vi "R30-Fpga.vi"() -> ()   [LabVIEW 2015]
uses:
  <vilib>/eio/EIONode/EIONode.xnode
  <vilib>/eio/EIOMethodNode/EIOMethodNode.xnode
  <vilib>/LabVIEW Targets/FPGA/cRIO/shared/nicrio_ModuleControls/nicrio_cRIO-9871_DataBitsEnum.ctl
  <vilib>/LabVIEW Targets/FPGA/cRIO/shared/nicrio_ModuleControls/nicrio_cRIO-9871_ParityEnum.ctl
  <vilib>/eio/EIOPropertyNode/EIOPropertyNode.xnode
  <vilib>/LabVIEW Targets/FPGA/cRIO/shared/nicrio_ModuleControls/nicrio_cRIO-9871_StopBitsEnum.ctl
  <vilib>/LabVIEW Targets/FPGA/cRIO/shared/nicrio_ModuleControls/nicrio_cRIO-9871_BaudRateEnum.ctl
  <vilib>/rvi/Analysis/measure/dc-rms/XNode/niFpgaDC-RMS.xnode
  <vilib>/rvi/eio/common/nirviEmuTemplateMethod_errors.vi
  <vilib>/Platform/TimedLoop/XDataNode/wakeup.ctl
  <vilib>/Platform/TimedLoop/XDataNode/XDNodeRunTimeDep.lvlib
  <vilib>/Platform/TimedLoop/XDataNode/nitl_modes.ctl
  <vilib>/Platform/TimedLoop/XDataNode/timing_clust.ctl
  <vilib>/Platform/TimedLoop/XDataNode/XDataNode.xnode
  <vilib>/rvi/FXPMathLib/basic elements/FxpIntAccumulator/XNode/nifxpmath_IntAccumulator.xnode
  <vilib>/rvi/FXPMathLib/FxpMul/XNode/nifxpmath_Multiplier.xnode
  <vilib>/rvi/Analysis/common/codeGenErrors/XNode/niFpgaXNodeCodeGenErrorHandle.vi
  <vilib>/rvi/FXPMathLib/basic elements/FxpIntAccumulator/simVIs/DllFxpIntAccumulator_sub.vi
  <vilib>/rvi/FXPMathLib/basic elements/FxpIntAccumulator/subVIs/nifxpmath_IntAccumulator_SimConfig.ctl
  <vilib>/rvi/FXPMathLib/sim/FxpSim.dll
  <vilib>/rvi/eio/common/nirviEmuTemplatePropertyGet_errors.vi
  <vilib>/rvi/eio/common/nirviEmuTemplatePropertyGet_noerrors.vi
  <vilib>/rvi/eio/common/nirviEmuTemplatePropertySet_errors.vi
  <vilib>/rvi/eio/common/nirviEmuTemplatePropertySet_noerrors.vi
  <vilib>/LabVIEW Targets/FPGA/cRIO/shared/nicrio_ModuleControls/nicrio_cRIO-9871_LineStateEnum.ctl
panel:
  out "analog readback":fxp<+/-,26,5>[](array[numeric]) format="%.23g"
  out "switch image ion gauge":u8[](array[numeric])
  out "Time since repurge":u8[](array[numeric])
  out "1st stage temp(k)":u8[](array[numeric])
  out "2nd stage":u8[](array[numeric])
  out "Time since pump on":u8[](array[numeric])
  out "Pump On":u8[](array[numeric])
  out "R30 ESA Convectron  1":u8[](array[numeric])
  out "R30 ESA Ion gauge 1":u8[](array[numeric])
  out "R30 Detector Convectron  1":u8[](array[numeric])
  out "R30 Detector Ion gauge 1":u8[](array[numeric])
  in  "y steerer magnet":fxp<+/-,20,5> format="%.17g"
  in  "analog output":fxp<+/-,64,32>[](array[numeric])=[0.0, 0.0, 0.0, 0.0, 0.0, 0.0, 0.0]
  out "Switch Ap IN":bool
  out "Switch Ap OUT2":bool
  out "Det Ap OUT":bool
  out "Det Ap IN":bool
  out "Detector  FC IN":bool
  out "Detector FC OUT":bool
  out "Switch magnet FC OUT":bool
  out "Switch magnet FC IN":bool
  in  "Switch magnet ap":bool
  in  "Detector AP":bool
  in  "Detector FC":bool
  in  "Switch magnet FC":bool
  out "Timed Out":bool
  out "Switch object tesla meter":u8[](array[numeric])
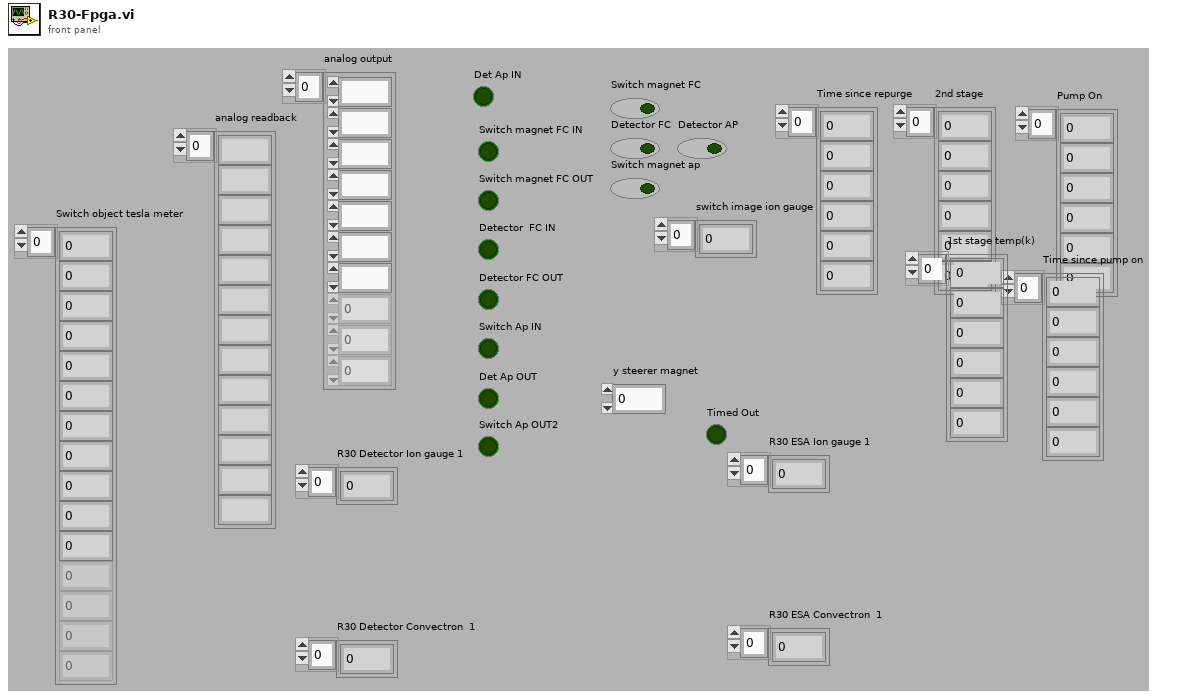
[diagram p1: front panel]
types:
  T1 = typedef "nicrio_cRIO-9871_StopBitsEnum.ctl" = enum8{"1", "1.5", "2"}
  T2 = typedef "nicrio_cRIO-9871_ParityEnum.ctl" = enum8{"None", "Odd", "Even", "Mark", "Space"}
  T3 = typedef "nicrio_cRIO-9871_DataBitsEnum.ctl" = enum8{"5", "6", "7", "8"}
  T4 = typedef "nicrio_cRIO-9871_BaudRateEnum.ctl" = enum16{"75 bps", "110 bps", "134 bps", "150 bps", "300 bps", "600 bps", "1200 bps", "1800 bps", "2400 bps", "4800 bps", "7200 bps", "9600 bps", "14.4 kbps", "19.2 kbps", "28.8 kbps", "38.4 kbps", "57.6 kbps", "115.2 kbps", "230.4 kbps", "460.8 kbps", "921.6 kbps"}
  T5 = typedef "XDNodeRunTimeDep.lvlib/timing_clust.ctl" = cluster{"Expected End [f-1]":u64, "Actual End [f-1]":u64, "Finished Late? [f-1]":bool, "Expected End [i-1]":u64, "Actual End [i-1]":u64, "Finished Late? [i-1]":bool, "Expected Start [i]":u64, "Actual Start [i]":u64, "Expected Start [f]":u64, "Actual Start [f]":u64, "Source Name":string, "Structure Name":string, "Period":i64, "Deadline":i64, "Offset":i64, "Start":i64, "Priority":i32, "Timeout":i32, "Mode":T6, "Wakeup Reason":T7, "Error":errorcluster, "Source Type":string, "Secondary Source Type":string, "Global End Time":u64, "Global Start Time":u64, "Frame Duration":u64, "Iteration Duration":u64, "Assigned CPU":i32, "I/O Scan Engine Mode":u32}
  T6 = typedef "XDNodeRunTimeDep.lvlib/nitl_modes.ctl" = enum32{"No Change", "Process missed periods, maintain original phase", "Discard missed periods, maintain original phase", "Process missed periods, ignore original phase", "Discard missed periods, ignore original phase"}
  T7 = typedef "XDNodeRunTimeDep.lvlib/wakeup.ctl" = enum32{"Normal", "Aborted", "Asynchronous wakeup", "Timing source error", "Timed loop error", "Timeout"}
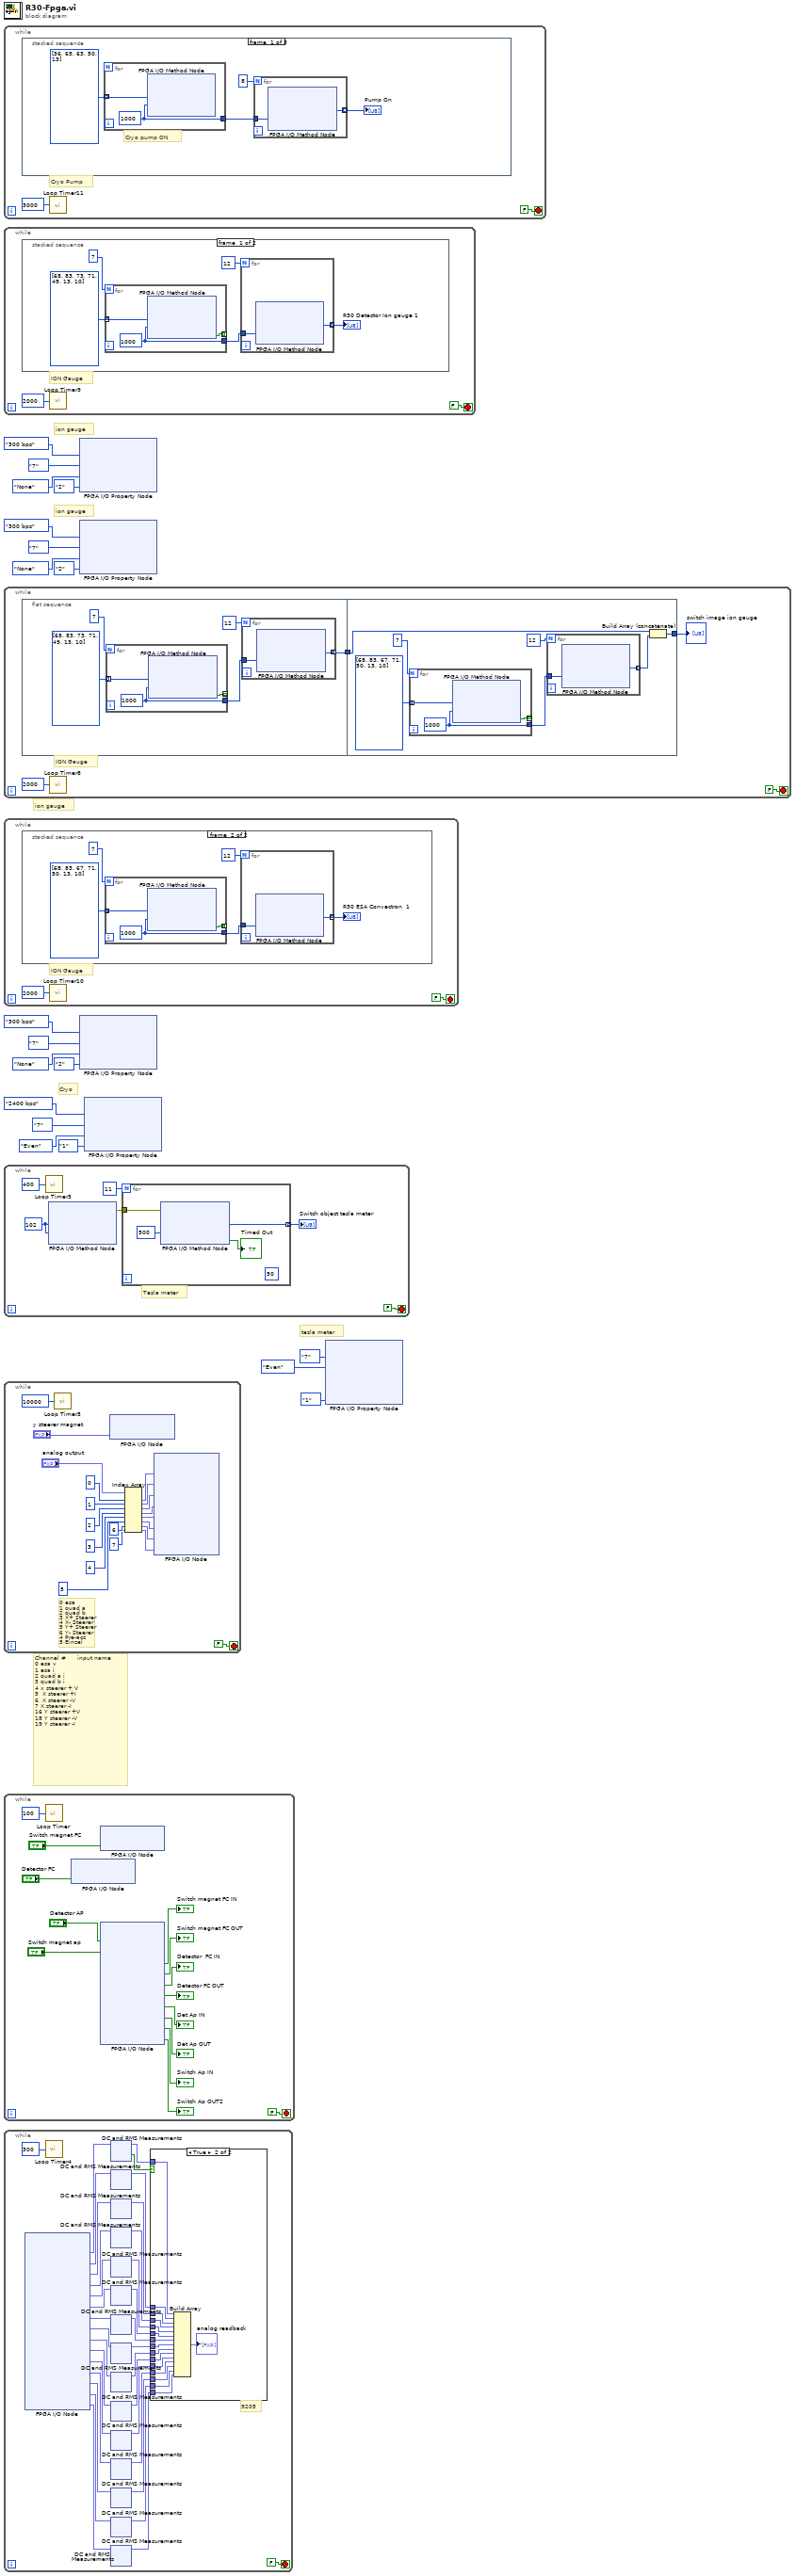
[diagram p0: block diagram]
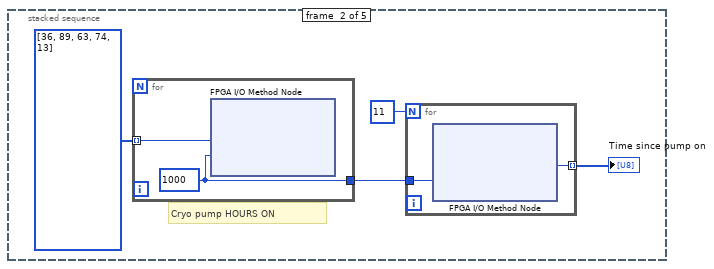
[diagram p2: hidden frame]
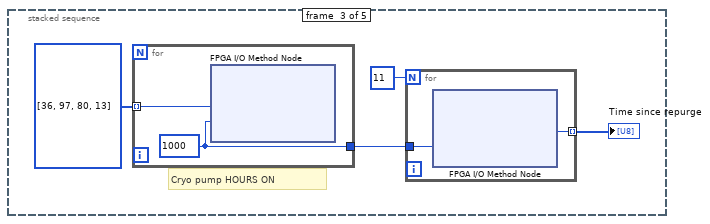
[diagram p3: hidden frame]
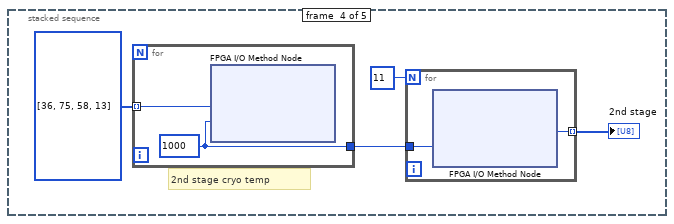
[diagram p4: hidden frame]
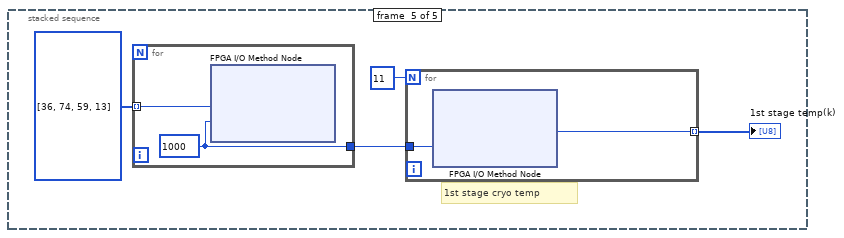
[diagram p5: hidden frame]
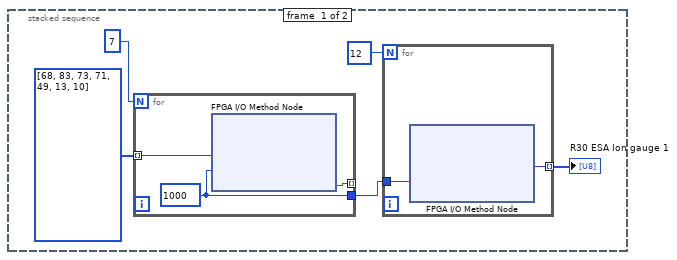
[diagram p6: hidden frame]
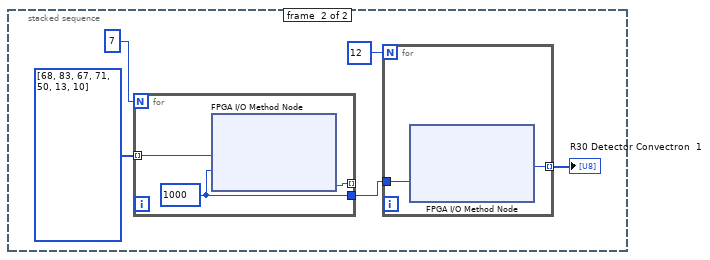
[diagram p7: hidden frame]
diagram:
  # "Channel #      input name\n0 esa v\n1 esa i\n2 quad a i\n3 quad b i\n4 x steerer + V\n5  X steerer +I\n6  X steerer -V\n7 X steerer -I\n16 Y steerer +V\n18 Y steerer -V\n19 Y steerer -I"
  # "tesla meter"
  # "Cryo"
  # "ion gauge"
  # "ion gauge"
  # "ion gauge"
  n1 = while {
    stop <- FALSE stop-if-true
    # "Cryo Pump"
    n2 = stacked-sequence {
      frame #0 {
        # "Cryo pump ON"
        n3 = for {
          tunnel: [w29] -> w25
          tunnel: u8[] [36, 65, 63, 50, 13] ("unsigned byte array") -> [w28] mode=indexing
          w29 = 1000 ("Timeout (ms)")
          n4 = xnode "FPGA I/O Method Node"("Data"=w28, "Timeout (ms)"=w29) -> ()  [unwired: 1 in, 2 out]
        }
        n5 = for {
          N: 8 -> [_]
          tunnel: w25 -> [w27]
          tunnel: [w26] -> w22 mode=indexing
          n6 = xnode "FPGA I/O Method Node"("Timeout (ms)"=w27) -> ("Data"=w26:u8)  [unwired: 1 in, 2 out]
        }
        "Pump On" <- w22
      }
      frame #1 {
        # "Cryo pump HOURS ON"
        n7 = for {
          tunnel: [w37] -> w33
          tunnel: u8[] [36, 89, 63, 74, 13] ("unsigned byte array") -> [w36] mode=indexing
          w37 = 1000 ("Timeout (ms)")
          n8 = xnode "FPGA I/O Method Node"("Data"=w36, "Timeout (ms)"=w37) -> ()  [unwired: 1 in, 2 out]
        }
        n9 = for {
          N: 11 -> [_]
          tunnel: w33 -> [w35]
          tunnel: [w34] -> w30 mode=indexing
          n10 = xnode "FPGA I/O Method Node"("Timeout (ms)"=w35) -> ("Data"=w34:u8)  [unwired: 1 in, 2 out]
        }
        "Time since pump on" <- w30
      }
      frame #2 {
        # "Cryo pump HOURS ON"
        n11 = for {
          tunnel: [w45] -> w41
          tunnel: u8[] [36, 97, 80, 13] ("unsigned byte array") -> [w44] mode=indexing
          w45 = 1000 ("Timeout (ms)")
          n12 = xnode "FPGA I/O Method Node"("Data"=w44, "Timeout (ms)"=w45) -> ()  [unwired: 1 in, 2 out]
        }
        n13 = for {
          N: 11 -> [_]
          tunnel: w41 -> [w43]
          tunnel: [w42] -> w38 mode=indexing
          n14 = xnode "FPGA I/O Method Node"("Timeout (ms)"=w43) -> ("Data"=w42:u8)  [unwired: 1 in, 2 out]
        }
        "Time since repurge" <- w38
      }
      frame #3 {
        # "2nd stage cryo temp"
        n15 = for {
          tunnel: [w53] -> w49
          tunnel: u8[] [36, 75, 58, 13] ("unsigned byte array") -> [w52] mode=indexing
          w53 = 1000 ("Timeout (ms)")
          n16 = xnode "FPGA I/O Method Node"("Data"=w52, "Timeout (ms)"=w53) -> ()  [unwired: 1 in, 2 out]
        }
        n17 = for {
          N: 11 -> [_]
          tunnel: w49 -> [w51]
          tunnel: [w50] -> w46 mode=indexing
          n18 = xnode "FPGA I/O Method Node"("Timeout (ms)"=w51) -> ("Data"=w50:u8)  [unwired: 1 in, 2 out]
        }
        "2nd stage" <- w46
      }
      frame #4 {
        # "1st stage cryo temp"
        n19 = for {
          tunnel: [w61] -> w57
          tunnel: u8[] [36, 74, 59, 13] ("unsigned byte array") -> [w60] mode=indexing
          w61 = 1000 ("Timeout (ms)")
          n20 = xnode "FPGA I/O Method Node"("Data"=w60, "Timeout (ms)"=w61) -> ()  [unwired: 1 in, 2 out]
        }
        n21 = for {
          N: 11 -> [_]
          tunnel: w57 -> [w59]
          tunnel: [w58] -> w54 mode=indexing
          n22 = xnode "FPGA I/O Method Node"("Timeout (ms)"=w59) -> ("Data"=w58:u8)  [unwired: 1 in, 2 out]
        }
        "1st stage temp(k)" <- w54
      }
    }
    n23 = call "Loop Timer11"("Count(mSec)"=u32 3000 ("Count(Ticks)")) -> ()  [unwired: 1 out]
  }
  n24 = while {
    stop <- FALSE stop-if-true
    # "ION Gauge"
    n25 = stacked-sequence {
      frame #0 {
        n26 = for {
          N: 7 -> [_]
          tunnel: [w73] -> w68
          tunnel: [w72] -> _ mode=indexing
          tunnel: u8[] [68, 83, 73, 71, 49, 13, 10] ("unsigned byte array") -> [w71] mode=indexing
          w73 = 1000 ("Timeout (ms)")
          n27 = xnode "FPGA I/O Method Node"("Data"=w71, "Timeout (ms)"=w73) -> ("Timed Out"=w72:bool)  [unwired: 1 in, 1 out]
        }
        n28 = for {
          N: 12 -> [_]
          tunnel: w68 -> [w70]
          tunnel: [w69] -> w64 mode=indexing
          n29 = xnode "FPGA I/O Method Node"("Timeout (ms)"=w70) -> ("Data"=w69:u8)  [unwired: 1 in, 2 out]
        }
        "R30 Detector Ion gauge 1" <- w64
      }
      frame #1 {
        n30 = for {
          N: 7 -> [_]
          tunnel: [w83] -> w78
          tunnel: [w82] -> _ mode=indexing
          tunnel: u8[] [68, 83, 67, 71, 50, 13, 10] ("unsigned byte array") -> [w81] mode=indexing
          w83 = 1000 ("Timeout (ms)")
          n31 = xnode "FPGA I/O Method Node"("Data"=w81, "Timeout (ms)"=w83) -> ("Timed Out"=w82:bool)  [unwired: 1 in, 1 out]
        }
        n32 = for {
          N: 12 -> [_]
          tunnel: w78 -> [w80]
          tunnel: [w79] -> w74 mode=indexing
          n33 = xnode "FPGA I/O Method Node"("Timeout (ms)"=w80) -> ("Data"=w79:u8)  [unwired: 1 in, 2 out]
        }
        "R30 Detector Convectron  1" <- w74
      }
    }
    n34 = call "Loop Timer9"("Count(mSec)"=u32 2000 ("Count(Ticks)")) -> ()  [unwired: 1 out]
  }
  n35 = while {
    stop <- FALSE stop-if-true
    # "ION Gauge"
    n36 = flat-sequence {
      tunnel: [w88] -> w85
      tunnel: w85 -> [w100]
      tunnel: [w98] -> w84
      frame #0 {
        n37 = for {
          N: 7 -> [_]
          tunnel: [w97] -> w92
          tunnel: [w96] -> _ mode=indexing
          tunnel: u8[] [68, 83, 73, 71, 49, 13, 10] ("unsigned byte array") -> [w95] mode=indexing
          w97 = 1000 ("Timeout (ms)")
          n38 = xnode "FPGA I/O Method Node"("Data"=w95, "Timeout (ms)"=w97) -> ("Timed Out"=w96:bool)  [unwired: 1 in, 1 out]
        }
        n39 = for {
          N: 12 -> [_]
          tunnel: w92 -> [w94]
          tunnel: [w93] -> w88 mode=indexing
          n40 = xnode "FPGA I/O Method Node"("Timeout (ms)"=w94) -> ("Data"=w93:u8)  [unwired: 1 in, 2 out]
        }
      }
      frame #1 {
        n41 = for {
          N: 7 -> [_]
          tunnel: [w109] -> w104
          tunnel: [w108] -> _ mode=indexing
          tunnel: u8[] [68, 83, 67, 71, 50, 13, 10] ("unsigned byte array") -> [w107] mode=indexing
          w109 = 1000 ("Timeout (ms)")
          n42 = xnode "FPGA I/O Method Node"("Data"=w107, "Timeout (ms)"=w109) -> ("Timed Out"=w108:bool)  [unwired: 1 in, 1 out]
        }
        n43 = for {
          N: 12 -> [_]
          tunnel: w104 -> [w106]
          tunnel: [w105] -> w99 mode=indexing
          n44 = xnode "FPGA I/O Method Node"("Timeout (ms)"=w106) -> ("Data"=w105:u8)  [unwired: 1 in, 2 out]
        }
        n45 = Build Array (concatenate)(w100, w99) -> (w98:u8[])
      }
    }
    n46 = call "Loop Timer8"("Count(mSec)"=u32 2000 ("Count(Ticks)")) -> ()  [unwired: 1 out]
    "switch image ion gauge" <- w84
  }
  n47 = while {
    stop <- FALSE stop-if-true
    # "ION Gauge"
    n48 = stacked-sequence {
      frame #0 {
        n49 = for {
          N: 7 -> [_]
          tunnel: [w121] -> w116
          tunnel: [w120] -> _ mode=indexing
          tunnel: u8[] [68, 83, 73, 71, 49, 13, 10] ("unsigned byte array") -> [w119] mode=indexing
          w121 = 1000 ("Timeout (ms)")
          n50 = xnode "FPGA I/O Method Node"("Data"=w119, "Timeout (ms)"=w121) -> ("Timed Out"=w120:bool)  [unwired: 1 in, 1 out]
        }
        n51 = for {
          N: 12 -> [_]
          tunnel: w116 -> [w118]
          tunnel: [w117] -> w112 mode=indexing
          n52 = xnode "FPGA I/O Method Node"("Timeout (ms)"=w118) -> ("Data"=w117:u8)  [unwired: 1 in, 2 out]
        }
        "R30 ESA Ion gauge 1" <- w112
      }
      frame #1 {
        n53 = for {
          N: 7 -> [_]
          tunnel: [w131] -> w126
          tunnel: [w130] -> _ mode=indexing
          tunnel: u8[] [68, 83, 67, 71, 50, 13, 10] ("unsigned byte array") -> [w129] mode=indexing
          w131 = 1000 ("Timeout (ms)")
          n54 = xnode "FPGA I/O Method Node"("Data"=w129, "Timeout (ms)"=w131) -> ("Timed Out"=w130:bool)  [unwired: 1 in, 1 out]
        }
        n55 = for {
          N: 12 -> [_]
          tunnel: w126 -> [w128]
          tunnel: [w127] -> w122 mode=indexing
          n56 = xnode "FPGA I/O Method Node"("Timeout (ms)"=w128) -> ("Data"=w127:u8)  [unwired: 1 in, 2 out]
        }
        "R30 ESA Convectron  1" <- w122
      }
    }
    n57 = call "Loop Timer10"("Count(mSec)"=u32 2000 ("Count(Ticks)")) -> ()  [unwired: 1 out]
  }
  n58 = while {
    stop <- FALSE stop-if-true
    w134 = u8 102 ("Data")
    # "Tesla meter"
    n59 = call "Loop Timer3"("Count(mSec)"=u32 400) -> ()  [unwired: 1 out]
    n60 = xnode "FPGA I/O Method Node"("Data"=w134, "Timeout (ms)"=w134) -> ("error out"=w133:errorcluster)  [unwired: 2 in, 2 out]
    n61 = for {
      N: 11 ("Numeric 3") -> [_]
      tunnel: [w139] -> w135 mode=indexing
      tunnel: w133 -> [w138]
      (unwired) 50 ("Timeout")
      n62 = xnode "FPGA I/O Method Node"("error in"=w138, "Timeout (ms)"=500) -> ("Data"=w139:u8, "Timed Out"=→"Timed Out":bool)  [unwired: 1 in, 2 out]
    }
    "Switch object tesla meter" <- w135
  }
  n63 = while {
    stop <- FALSE stop-if-true
    # "0 esa\n1 quad a\n2 quad b\n3 X+ Steerer\n4 X- Steerer\n5 Y+ Steerer\n6 Y- Steerer\n4 Pre-acc\n5 Einzel"
    n64 = call "Loop Timer5"("Count(Ticks)"=u32 10000 ("Count(mSec)")) -> ()  [unwired: 1 out]
    n65 = xnode "FPGA I/O Node"("Mod6/AO0"="y steerer magnet") -> ()  [unwired: 1 in, 1 out]
    n66 = Index Array(array="analog output", index #1=0 ("index"), index #2=1 ("index"), index #3=2 ("index"), index #4=3 ("index"), index #5=4 ("index"), index #6=5 ("index"), index #7=6 ("index"), index #8=7 ("index")) -> (element #1=w149:fxp<+/-,64,32>, element #2=w148:fxp<+/-,64,32>, element #3=w147:fxp<+/-,64,32>, element #4=w146:fxp<+/-,64,32>, element #5=w145:fxp<+/-,64,32>, element #6=w144:fxp<+/-,64,32>, element #7=w143:fxp<+/-,64,32>, element #8=w142:fxp<+/-,64,32>)
    n67 = xnode "FPGA I/O Node"("Mod1/AO0"=w149, "Mod1/AO1"=w148, "Mod1/AO2"=w147, "Mod1/AO3"=w146, "Mod1/AO4"=w145, "Mod1/AO5"=w144, "Mod1/AO6"=w143, "Mod1/AO7"=w142) -> ()  [unwired: 8 in, 8 out]
  }
  n68 = while {
    stop <- FALSE stop-if-true
    n69 = call "Loop Timer"("Count(mSec)"=u32 100 ("Count(uSec)")) -> ()  [unwired: 1 out]
    n70 = xnode "FPGA I/O Node"("Mod8/CH1"="Detector FC") -> ()  [unwired: 1 in, 1 out]
    n71 = xnode "FPGA I/O Node"("Mod8/CH0"="Switch magnet FC") -> ()  [unwired: 1 in, 1 out]
    n72 = xnode "FPGA I/O Node"("Mod8/CH2"="Detector AP", "Mod8/CH3"="Switch magnet ap") -> ("Mod7/DI0"=→"Switch magnet FC IN":bool, "Mod7/DI1"=→"Switch magnet FC OUT":bool, "Mod7/DI2"=→"Detector  FC IN":bool, "Mod7/DI3"=→"Detector FC OUT":bool, "Mod7/DI4"=→"Det Ap IN":bool, "Mod7/DI5"=→"Det Ap OUT":bool, "Mod7/DI6"=→"Switch Ap IN":bool, "Mod7/DI7"=→"Switch Ap OUT2":bool)  [unwired: 10 in, 10 out]
  }
  n73 = while {
    stop <- FALSE stop-if-true
    # "9205"
    n74 = xnode "FPGA I/O Node"() -> ("Mod2/AI0"=w205:fxp<+/-,26,5>, "Mod2/AI1"=w203:fxp<+/-,26,5>, "Mod2/AI2"=w201:fxp<+/-,26,5>, "Mod2/AI3"=w199:fxp<+/-,26,5>, "Mod2/AI4"=w197:fxp<+/-,26,5>, "Mod2/AI5"=w195:fxp<+/-,26,5>, "Mod2/AI6"=w193:fxp<+/-,26,5>, "Mod2/AI7"=w191:fxp<+/-,26,5>, "Mod2/AI16"=w189:fxp<+/-,26,5>, "Mod2/AI17"=w187:fxp<+/-,26,5>, "Mod2/AI18"=w185:fxp<+/-,26,5>, "Mod2/AI19"=w183:fxp<+/-,26,5>, "Mod2/AI20"=w181:fxp<+/-,26,5>, "Mod2/AI21"=w179:fxp<+/-,26,5>, "Mod2/AI22"=w177:fxp<+/-,26,5>)  [unwired: 15 in, 15 out]
    n75 = call "Loop Timer4"("Count(Ticks)"=u32 300) -> ()  [unwired: 1 out]
    n76 = xnode "DC and RMS Measurements"("input data"=w205) -> ("DC"=w204:fxp<+/-,26,5>, "output valid"=w206:bool)  [unwired: 1 in]
    n77 = xnode "DC and RMS Measurements"("input data"=w203) -> ("DC"=w202:fxp<+/-,26,5>)  [unwired: 1 in, 1 out]
    n78 = xnode "DC and RMS Measurements"("input data"=w201) -> ("DC"=w200:fxp<+/-,26,5>)  [unwired: 1 in, 1 out]
    n79 = xnode "DC and RMS Measurements"("input data"=w199) -> ("DC"=w198:fxp<+/-,26,5>)  [unwired: 1 in, 1 out]
    n80 = xnode "DC and RMS Measurements"("input data"=w197) -> ("DC"=w196:fxp<+/-,26,5>)  [unwired: 1 in, 1 out]
    n81 = xnode "DC and RMS Measurements"("input data"=w195) -> ("DC"=w194:fxp<+/-,26,5>)  [unwired: 1 in, 1 out]
    n82 = xnode "DC and RMS Measurements"("input data"=w193) -> ("DC"=w192:fxp<+/-,26,5>)  [unwired: 1 in, 1 out]
    n83 = xnode "DC and RMS Measurements"("input data"=w191) -> ("DC"=w190:fxp<+/-,26,5>)  [unwired: 1 in, 1 out]
    n84 = xnode "DC and RMS Measurements"("input data"=w189) -> ("DC"=w188:fxp<+/-,26,5>)  [unwired: 1 in, 1 out]
    n85 = xnode "DC and RMS Measurements"("input data"=w187) -> ("DC"=w186:fxp<+/-,26,5>)  [unwired: 1 in, 1 out]
    n86 = xnode "DC and RMS Measurements"("input data"=w185) -> ("DC"=w184:fxp<+/-,26,5>)  [unwired: 1 in, 1 out]
    n87 = xnode "DC and RMS Measurements"("input data"=w183) -> ("DC"=w182:fxp<+/-,26,5>)  [unwired: 1 in, 1 out]
    n88 = xnode "DC and RMS Measurements"("input data"=w181) -> ("DC"=w180:fxp<+/-,26,5>)  [unwired: 1 in, 1 out]
    n89 = xnode "DC and RMS Measurements"("input data"=w179) -> ("DC"=w178:fxp<+/-,26,5>)  [unwired: 1 in, 1 out]
    n90 = xnode "DC and RMS Measurements"("input data"=w177) -> ("DC"=w176:fxp<+/-,26,5>)  [unwired: 1 in, 1 out]
    n91 = case shown="True" w206 {
      tunnel: w204 -> [_ w383]
      tunnel: w202 -> [_ w382]
      tunnel: w200 -> [_ w381]
      tunnel: w198 -> [_ w380]
      tunnel: w196 -> [_ w379]
      tunnel: w194 -> [_ w378]
      tunnel: w192 -> [_ w377]
      tunnel: w190 -> [_ w376]
      tunnel: w188 -> [_ w375]
      tunnel: w186 -> [_ w374]
      tunnel: w184 -> [_ w373]
      tunnel: w182 -> [_ w372]
      tunnel: w180 -> [_ w371]
      tunnel: w178 -> [_ w370]
      tunnel: w176 -> [_ w369]
      frame False {
      }
      frame True {
        n92 = Build Array(w383, w382, w381, w380, w379, w378, w377, w376, w375, w374, w373, w372, w371, w370, w369) -> (→"analog readback":fxp<+/-,26,5>[])
      }
    }
  }
  n93 = xnode "FPGA I/O Property Node"("Baud Rate"=nicrio_cRIO-9871_BaudRateEnum."300 bps", "Data Bits"=nicrio_cRIO-9871_DataBitsEnum."7", "Parity"=nicrio_cRIO-9871_ParityEnum."None", "Stop Bits"=nicrio_cRIO-9871_StopBitsEnum."2") -> ()  [unwired: 1 in, 1 out]
  n94 = xnode "FPGA I/O Property Node"("Baud Rate"=nicrio_cRIO-9871_BaudRateEnum."300 bps", "Data Bits"=nicrio_cRIO-9871_DataBitsEnum."7", "Parity"=nicrio_cRIO-9871_ParityEnum."None", "Stop Bits"=nicrio_cRIO-9871_StopBitsEnum."2") -> ()  [unwired: 1 in, 1 out]
  n95 = xnode "FPGA I/O Property Node"("Baud Rate"=nicrio_cRIO-9871_BaudRateEnum."300 bps", "Data Bits"=nicrio_cRIO-9871_DataBitsEnum."7", "Parity"=nicrio_cRIO-9871_ParityEnum."None", "Stop Bits"=nicrio_cRIO-9871_StopBitsEnum."2") -> ()  [unwired: 1 in, 1 out]
  n96 = xnode "FPGA I/O Property Node"("Baud Rate"=nicrio_cRIO-9871_BaudRateEnum."2400 bps", "Data Bits"=nicrio_cRIO-9871_DataBitsEnum."7", "Parity"=nicrio_cRIO-9871_ParityEnum."Even", "Stop Bits"=nicrio_cRIO-9871_StopBitsEnum."1") -> ()  [unwired: 1 in, 1 out]
  n97 = xnode "FPGA I/O Property Node"("Data Bits"=nicrio_cRIO-9871_DataBitsEnum."7", "Parity"=nicrio_cRIO-9871_ParityEnum."Even", "Stop Bits"=nicrio_cRIO-9871_StopBitsEnum."1") -> ()  [unwired: 2 in, 2 out]
